vi "AssigningButtons_171213.vi"(11 "Input":string[][](array[string])) -> (2 "Cancel Button 2":bool, 3 "outputarray":string[][](array[string]))   [LabVIEW 2016]
panel:
  in  "Tab Control":enum32{"Page 1", "Page 2"}(tab)
  in  "Cancel Button":bool
  in  "OK Button":bool
  in  "KeyboardShortCuts":i32(listbox)
  in  "OK":bool
  in  "Behaviour":string
  in  "Button":string
  in  "Stop":bool
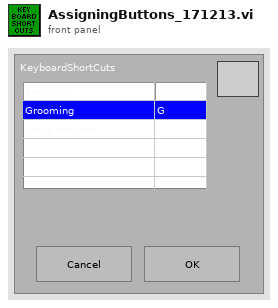
[diagram p1: front panel]
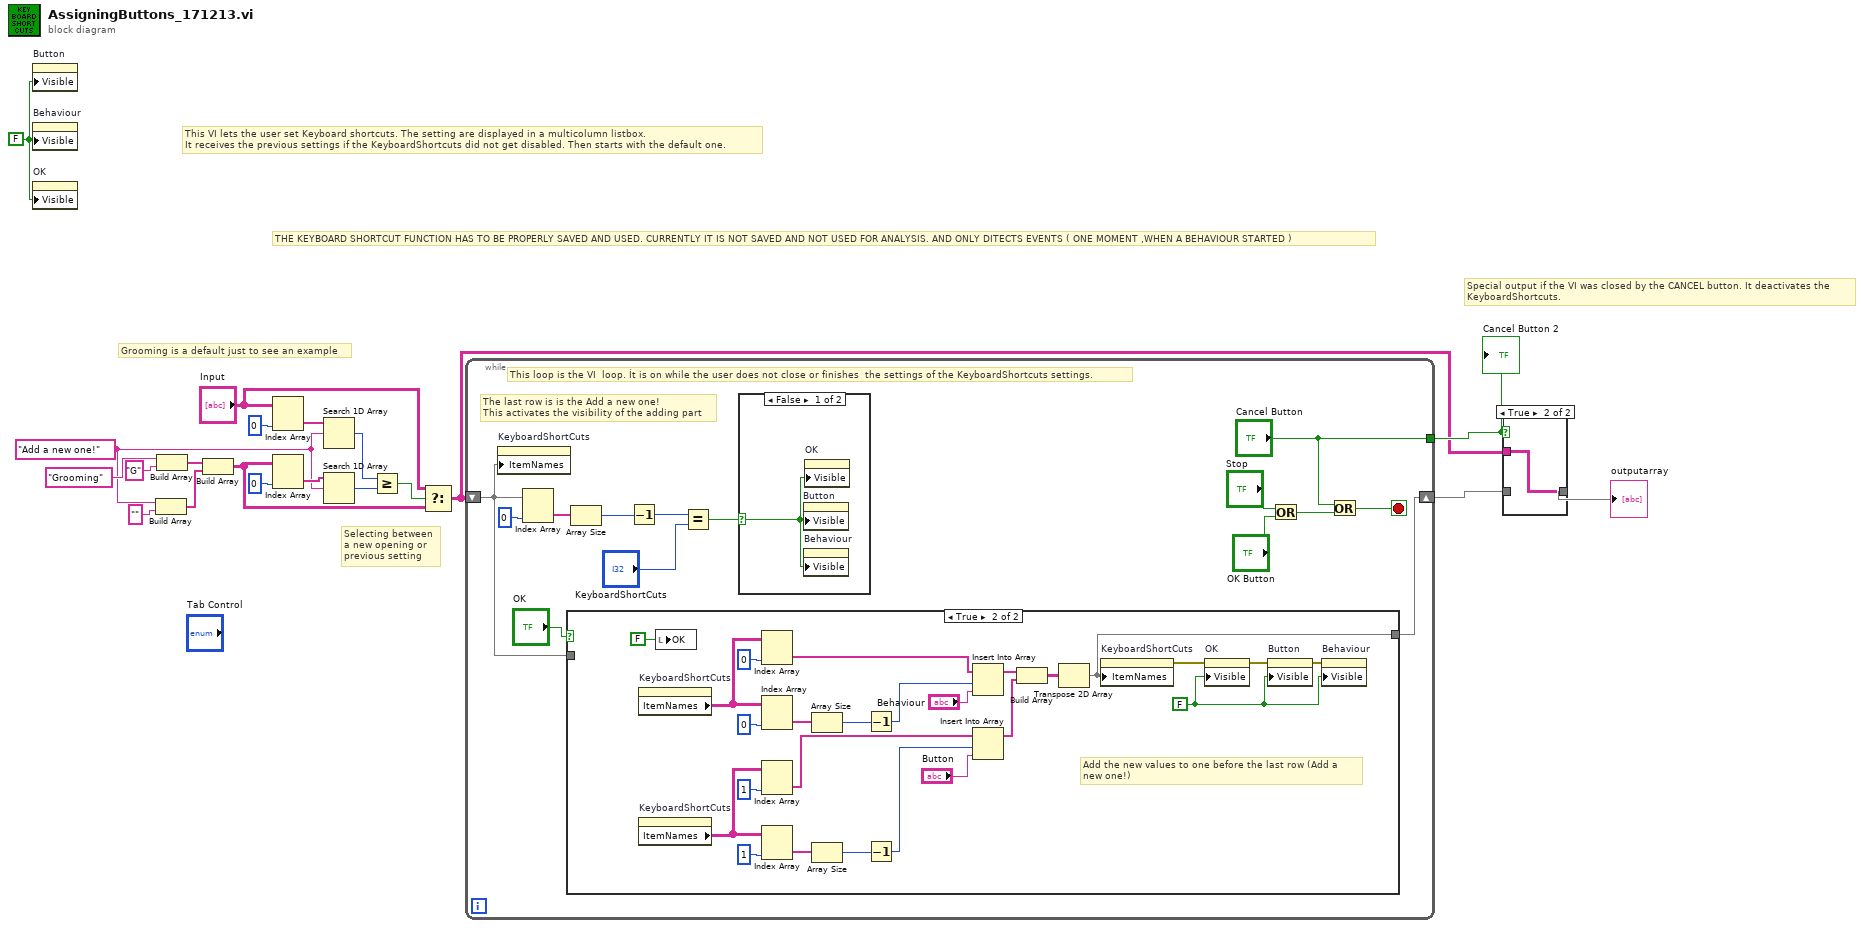
[diagram p0: block diagram]
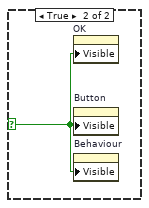
[diagram p3: hidden frame]
diagram:
  w5 = FALSE ("Visible")
  w10 = "Add a new one!"
  # "Special output if the VI was closed by the CANCEL button. It deactivates the\nKeyboardShortcuts."
  # "Selecting between\na new opening or \nprevious setting"
  # "THE KEYBOARD SHORTCUT FUNCTION HAS TO BE PROPERLY SAVED AND USED. CURRENTLY IT IS NOT SAVED AND NOT USED FOR ANALYSIS. AND ONLY DITECTS EVENTS ( ONE MOMENT ,WHEN A BEHAVIOUR STARTED )"
  # "This VI lets the user set Keyboard shortcuts. The setting are displayed in a multicolumn listbox.\nIt receives the previous settings if the KeyboardShortcuts did not get disabled. Then starts with the default one."
  # "Grooming is a default just to see an example"
  n1 = property on="Button" class="Str"("Visible"=w5) -> ()  [unwired: 2 in, 2 out]
  n2 = property on="Behaviour" class="Str"("Visible"=w5) -> ()  [unwired: 2 in, 2 out]
  n3 = property on="OK" class="Bool (strict)"("Visible"=w5) -> ()  [unwired: 2 in, 2 out]
  n4 = Build Array(w10, "" ("element")) -> (w20:string[])
  n5 = Build Array("Grooming", "G" ("element")) -> (w18:string[])
  n6 = Build Array(w18, w20) -> (w6:string[][])
  n7 = Index Array(array="Input", index (col)=0 ("disabled index (col)")) -> (element=w8:string[])  [unwired: 1 in]
  n8 = Index Array(array=w6, index (col)=0 ("disabled index (col)")) -> (element=w13:string[])  [unwired: 1 in]
  n9 = Search 1D Array(1D array=w8, element=w10) -> (index of element=w11:i32)  [unwired: 1 in]
  n10 = Search 1D Array(1D array=w13, element=w10) -> (index of element=w12:i32)  [unwired: 1 in]
  n11 = Greater Or Equal?(x=w11, y=w12) -> (x >= y?=w9:bool)
  n12 = Select(t="Input", s=w9, f=w6) -> (s? t:f=w1:string[][])
  n13 = while {
    shift-right: [w34] -> w2
    shift-left: w1 -> [w27]
    tunnel: ["Cancel Button"] -> w4
    stop <- w23 stop-if-true
    # "The last row is is the Add a new one!\nThis activates the visibility of the adding part"
    # "This loop is the VI  loop. Ít is on while the user does not close or finishes  the settings of the KeyboardShortcuts settings."
    n14 = property on="KeyboardShortCuts" class="MCListbox (strict)"("ItemNames"=w27) -> ()  [unwired: 2 in, 2 out]
    n15 = Index Array(array=w27, index (col)=0 ("index (row)")) -> (element=w30:string[])  [unwired: 1 in]
    n16 = case shown="True" "OK" {
      tunnel: [w37 w40] -> w34
      tunnel: w27 -> [w37 _]
      frame False {
      }
      frame True {
        w62 = FALSE ("Visible")
        # "Add the new values to one before the last row (Add a \nnew one!)"
        n17 = property on="KeyboardShortCuts" class="MCListbox (strict)"() -> ("ItemNames"=w44:string[][])  [unwired: 2 in, 2 out]
        n18 = property on="KeyboardShortCuts" class="MCListbox (strict)"() -> ("ItemNames"=w48:string[][])  [unwired: 2 in, 2 out]
        n19 = local write "OK"(FALSE ("OK")) -> ()
        n20 = Index Array(array=w44, index (col)=0 ("index (row)")) -> (element=w45:string[])  [unwired: 1 in]
        n21 = Index Array(array=w44, index (col)=0 ("index (row)")) -> (element=w43:string[])  [unwired: 1 in]
        n22 = Index Array(array=w48, index (col)=1 ("index (row)")) -> (element=w51:string[])  [unwired: 1 in]
        n23 = Index Array(array=w48, index (col)=1 ("index (row)")) -> (element=w49:string[])  [unwired: 1 in]
        n24 = Array Size(array=w43) -> (size(s)=w42:i32)
        n25 = Array Size(array=w49) -> (size(s)=w50:i32)
        n26 = Decrement(x=w42) -> (x-1=w46:i32)
        n27 = Decrement(x=w50) -> (x-1=w47:i32)
        n28 = Insert Into Array(array=w45, index=w46, new element="Behaviour") -> (w56:string[])
        n29 = Insert Into Array(array=w51, index=w47, new element="Button") -> (w57:string[])
        n30 = Build Array(w56, w57) -> (w58:string[][])
        n31 = Transpose 2D Array(2D array=w58) -> (transposed array=w40:string[][])
        n32 = property on="KeyboardShortCuts" class="MCListbox (strict)"("ItemNames"=w40) -> (error out=w59:errorcluster)  [unwired: 2 in, 1 out]
        n33 = property on="OK" class="Bool (strict)"(error in=w59, "Visible"=w62) -> (error out=w60:errorcluster)  [unwired: 1 in, 1 out]
        n34 = property on="Button" class="Str"(error in=w60, "Visible"=w62) -> (error out=w61:errorcluster)  [unwired: 1 in, 1 out]
        n35 = property on="Behaviour" class="Str"(error in=w61, "Visible"=w62) -> ()  [unwired: 1 in, 2 out]
      }
    }
    n36 = Array Size(array=w30) -> (size(s)=w32:i32)
    n37 = Decrement(x=w32) -> (x-1=w28:i32)
    n38 = Equal?(x=w28, y="KeyboardShortCuts") -> (x = y?=w31:bool)
    n39 = case shown="False" w31 {
      selector: w31 -> [w35 w36]
      frame False {
        n40 = property on="Button" class="Str"("Visible"=w35) -> ()  [unwired: 2 in, 2 out]
        n41 = property on="Behaviour" class="Str"("Visible"=w35) -> ()  [unwired: 2 in, 2 out]
        n42 = property on="OK" class="Bool (strict)"("Visible"=w35) -> ()  [unwired: 2 in, 2 out]
      }
      frame True {
        n43 = property on="OK" class="Bool (strict)"("Visible"=w36) -> ()  [unwired: 2 in, 2 out]
        n44 = property on="Button" class="Str"("Visible"=w36) -> ()  [unwired: 2 in, 2 out]
        n45 = property on="Behaviour" class="Str"("Visible"=w36) -> ()  [unwired: 2 in, 2 out]
      }
    }
    n46 = Or(x="Stop", y="OK Button") -> (x .or. y?=w24:bool)
    n47 = Or(x="Cancel Button", y=w24) -> (x .or. y?=w23:bool)
  }
  "Cancel Button 2" <- w4
  n48 = case shown="True" w4 {
    tunnel: [w63 w64] -> w3
    tunnel: w2 -> [w63 _]
    tunnel: w1 -> [_ w64]
    frame False {
    }
    frame True {
    }
  }
  "outputarray" <- w3
